vi "Save As Measurement Service Helpers.vi"(8 "error in":errorcluster, 11 "Project ref":refnum<vi>) -> (0 "error out":errorcluster)   [LabVIEW 2020, in "MeasurementService Editor.lvlib"]
uses:
  MeasurementService Editor.lvlib
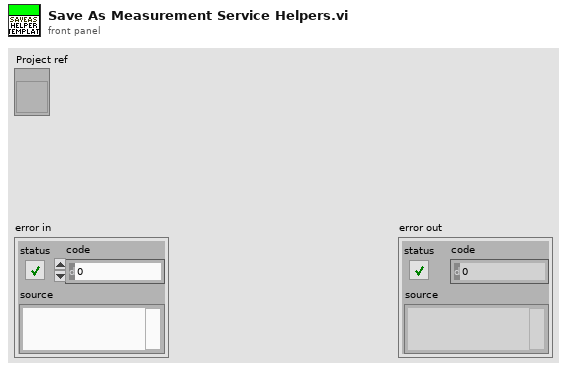
[diagram p1: front panel]
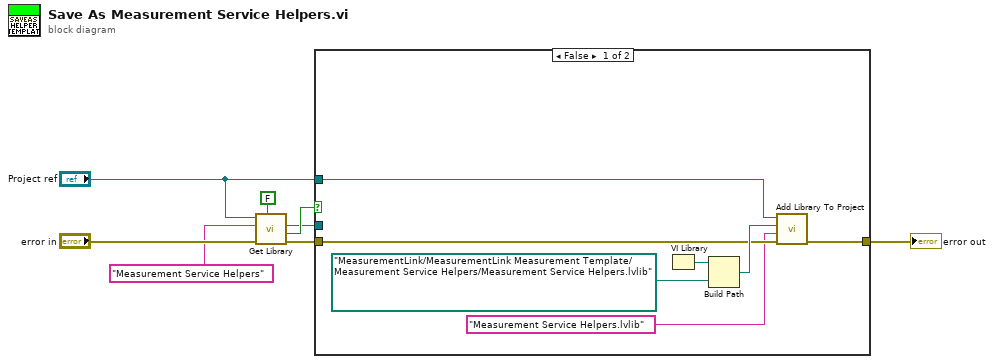
[diagram p0: block diagram]
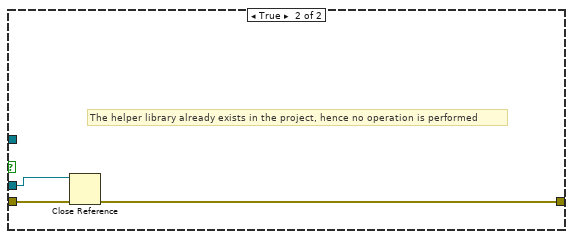
[diagram p2: hidden frame]
diagram:
  n1 = call "Get Library.vi"("Error if not Found (T)"=FALSE, "error in (no error)"="error in", "Measurement Service Name"="Measurement Service Helpers", "Project in"="Project ref") -> ("error out"=w6:errorcluster, "Found"=w4:bool, "Measurement Library Item"=w2:refnum<vi>)  [unwired: 5 in]
  n2 = case shown="False" w4 {
    tunnel: [w15 w17] -> w7
    tunnel: w6 -> [w11 w18]
    tunnel: w2 -> [_ w16]
    tunnel: "Project ref" -> [w10 _]
    frame False {
      n3 = VI Library() -> (path=w14:path)
      n4 = Build Path(base path=w14, name or relative path=path "MeasurementLink/MeasurementLink Measurement Template/Measurement Service Helpers/Measurement Service Helpers.lvlib" ("Library Path")) -> (appended path=w12:path)
      n5 = call "Add Library To Project.vi"("error in"=w11, "New Library Name"="Measurement Service Helpers.lvlib", "Library Path"=w12, "Project ref"=w10) -> ("error out"=w15:errorcluster)  [unwired: 7 in]
    }
    frame True {
      # "The helper library already exists in the project, hence no operation is performed"
      n6 = Close Reference(reference=w16, error in (no error)=w18) -> (error out=w17:errorcluster)
    }
  }
  "error out" <- w7
